vi "HTSuperProReadDigital.vi"(0 "Mask":u8=255 format="%x", 3 "NXT":T1={"error"={"status"=FALSE, "code"=0, "source"=""}, "address"="", "NXT #"=-1, "Show Error"=TRUE, "Connection"=4} {"Connection" items=["USB", "Bluetooth", "USB then Bluetooth", "Last Connection", "Preference"]}, 4 "Port":T2 items=["Port 1", "Port 2", "Port 3", "Port 4"]) -> (2 "Digital Value":u8, 5 "NXT":T1={"error"={"status"=FALSE, "code"=0, "source"=""}, "address"="", "NXT #"=-1, "Show Error"=TRUE, "Connection"=4} {"Connection" items=["USB", "Bluetooth", "USB then Bluetooth", "Last Connection", "Preference"]})   [LabVIEW 2009]
doc: "HiTechnic SuperPro - Read Digital Port\n\n<B>Inputs\nPort </B> is the port connected to the sensor. Port 1 is the default, but Port 2, Port 3, or Port 4 can also be selected.\n<B>NXT </B> connects to NXT terminal of previous VI to establish the flow of the program.\n<B>Mask </B> used to limit bits that are returned in the Digital Value. Only bits set to 1 in the mask are returned. (default is xFF)\n\n<B>Outputs\nNXT </B> wires to NXT terminal of next VI to establish the flow of the program.\n<B>Digital Value</B> result of reading the digital B7-B0 pins from the SuperPro."
uses:
  <vilib>/NXT/Block Support/NXT_InputPort.ctl
  <vilib>/NXT/Subs/LVHSConnector.ctl
  <vilib>/NXT/Block Support/HWPage.SensorType.ctl
  <vilib>/NXT/Block Support/HWPage.SensorMode.ctl
panel:
  # "HiTechnic SuperPro Prototype board VI\nRead Digital Port\n\nReads the digital port on the HiTechnic SuperPro board.  Use the Mask input to limit the bits that are returns.  Only bits set to 1 in the Mask are returns in the output digital Value.  If Mask is not specified, then all bits are returned.\n\n(c) HiTechnic 2011"
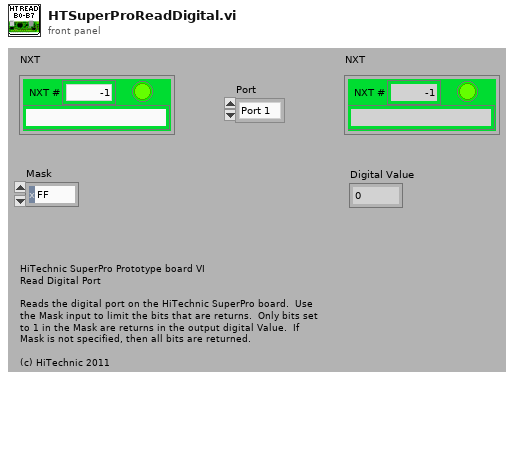
[diagram p1: front panel]
types:
  T1 = typedef "LVHSConnector.ctl" = cluster{"error":errorcluster, "address":string, "NXT #":i32, "Show Error":bool, "Connection":u16}
  T2 = typedef "NXT_InputPort.ctl" = u8
  T3 = typedef "HWPage.SensorType.ctl" = u8
  T4 = typedef "HWPage.SensorMode.ctl" = u8
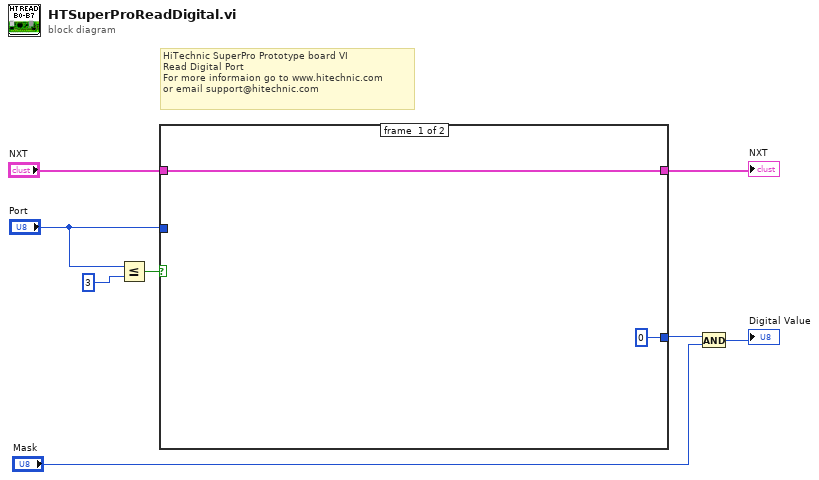
[diagram p0: block diagram]
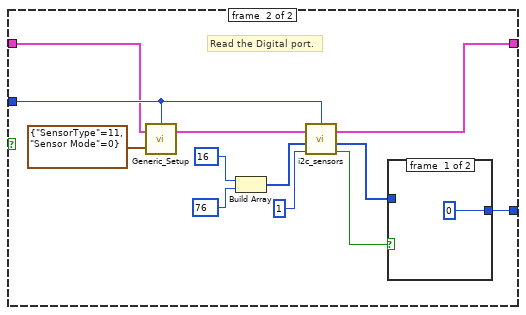
[diagram p2: hidden frame]
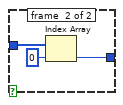
[diagram p3: hidden frame]
diagram:
  # "HiTechnic SuperPro Prototype board VI\nRead Digital Port\nFor more informaion go to www.hitechnic.com\nor email support@hitechnic.com"
  n1 = Less Or Equal?(x="Port", y=u8 3) -> (x <= y?=w4:bool)
  n2 = case shown="True" w4 {
    tunnel: "Port" -> [_ w21]
    tunnel: "NXT" -> [w9 w20]
    tunnel: [w9 w18] -> w6
    tunnel: [u8 0 w17] -> w3
    frame #0 {
    }
    frame #1 {
      # "Read the Digital port."
      n3 = call <vilib>:"Generic_Setup.vi"("Sensor Setup"=cluster{"SensorType":T3, "Sensor Mode":T4} {"SensorType"=11, "Sensor Mode"=0}, "NXT"=w20, "Port"=w21) -> ("NXT"=w19:T1)  [unwired: 1 out]
      n4 = Build Array(u8 16, u8 76) -> (w15:u8[])
      n5 = call <vilib>:"i2c_sensors.vi"("Return Length"=u8 1, "Bytes to Write"=w15, "NXT"=w19, "Port"=w21) -> ("Success?"=w13:bool, "Bytes read"=w12:u8[], "NXT"=w18:T1)  [unwired: 1 in]
      n6 = case shown="True" w13 {
        tunnel: w12 -> [_ w25]
        tunnel: [u8 0 w24] -> w17
        frame #0 {
        }
        frame #1 {
          n7 = Index Array(array=w25, index=0) -> (element=w24:u8)
        }
      }
    }
  }
  "NXT" <- w6
  n8 = And(x=w3, y="Mask") -> (x .and. y?=→"Digital Value":u8)
